vi "Destroy Queue.vi"(8 "error in (no error)":errorcluster, 11 "Message Queue in":refnum<class "Message Queue.lvclass">) -> (0 "error out":errorcluster, 2 "Remaining Elements":T1[](array[typedef]), 3 "Message Queue out":refnum<class "Message Queue.lvclass">)   [LabVIEW 2019, in "Network Interface.lvlib" / "Message Queue.lvclass"]
uses:
  <vilib>/gpm_packages/@cs/Network-Sink/Source/Network Interface/Message Queue/Message Queue.lvclass
  <vilib>/gpm_packages/@cs/Network-Sink/Source/Network Interface/Message Queue/Message Cluster.ctl
  <vilib>/gpm_packages/@cs/Network-Sink/Source/Network Interface/Message Queue/Message Queue.lvclass/Message Queue.ctl
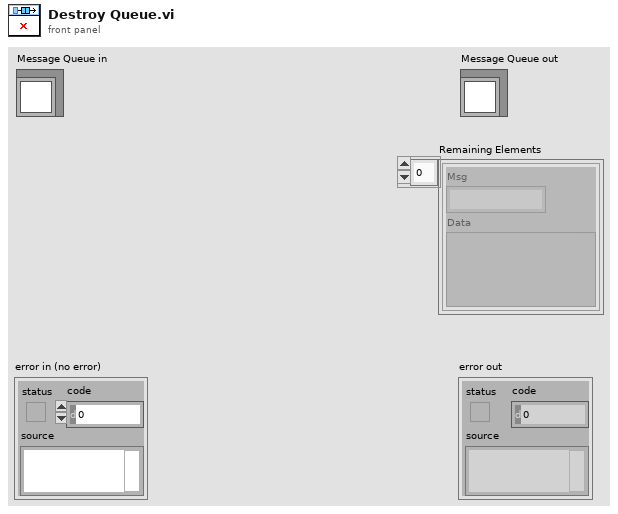
[diagram p1: front panel]
types:
  T1 = typedef "Network Interface.lvlib/Message Queue.lvclass/Message Cluster.ctl" = cluster{"Msg":string, "Data":variant}
  T2 = typedef "Network Sink.lvlib/Message Cluster.ctl" = cluster{"Msg":string, "Data":variant}
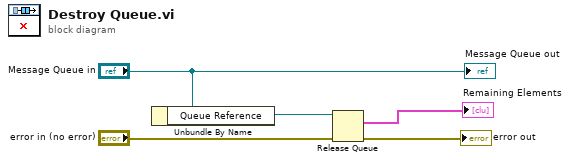
[diagram p0: block diagram]
diagram:
  n1 = Unbundle By Name("Message Queue in") -> ("Queue Reference"=w4:refnum<queue>)
  n2 = Release Queue(queue=w4, error in (no error)="error in (no error)") -> (remaining elements=→"Remaining Elements":T2[], error out=→"error out":errorcluster)  [unwired: 1 in, 1 out]
  "Message Queue out" <- "Message Queue in"
